vi "Inches to Shooter Angle.vi"(11 "distance (in)":dbl) -> (3 "arm angle":dbl)   [LabVIEW 2015]
uses:
  <vilib>/Analysis/NI_AALPro.lvlib
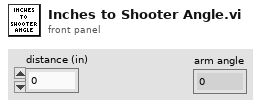
[diagram p1: front panel]
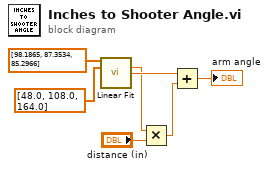
[diagram p0: block diagram]
diagram:
  n1 = call <vilib>:"Linear Fit.vi"("Y"=dbl[] [98.1865, 87.3534, 85.2966] ("X"), "X"=dbl[] [48.0, 108.0, 164.0] ("Y")) -> ("slope"=w4:dbl, "intercept"=w5:dbl)  [unwired: 9 in, 3 out]
  n2 = Multiply(x=w4, y="distance (in)") -> (x*y=w6:dbl)
  n3 = Add(x=w5, y=w6) -> (x+y=→"arm angle":dbl)
